vi "BMP180 Read.vi"(8 "error in (no error)":errorcluster, 9 "BMP180 Config":T1={"I2C"={"Slave Address"=64, "Channel"=0}, "Mode"=enum."Ultra Low Power", "Cal Coefs"={"AC1"={"Addr:"=170, "Val:"=0}, "AC2"={"Addr:"=172, "Val:"=0}, "AC3"={"Addr:"=174, "Val:"=0}, "AC4"={"Addr:"=176, "Val:"=0}, "AC5"={"Addr:"=178, "Val:"=0}, "AC6"={"Addr:"=180, "Val:"=0}, "B1"={"Addr:"=182, "Val:"=0}, "B2"={"Addr:"=184, "Val:"=0}, "MB"={"Addr:"=186, "Val:"=0}, "MC"={"Addr:"=188, "Val:"=0}, "MD"={"Addr:"=190, "Val:"=0}}, "Online"=FALSE} {"I2C"."Slave Address" format="%.0x"; "Cal Coefs"."MD"."Val:" format="%04x"; "Cal Coefs"."MD"."Addr:" format="%02x"; "Cal Coefs"."MC"."Val:" format="%04x"; "Cal Coefs"."MC"."Addr:" format="%02x"; "Cal Coefs"."MB"."Val:" format="%04x"; "Cal Coefs"."MB"."Addr:" format="%02x"; "Cal Coefs"."B2"."Val:" format="%04x"; "Cal Coefs"."B2"."Addr:" format="%02x"; "Cal Coefs"."B1"."Val:" format="%04x"; "Cal Coefs"."B1"."Addr:" format="%02x"; "Cal Coefs"."AC6"."Val:" format="%04x"; "Cal Coefs"."AC6"."Addr:" format="%02x"; "Cal Coefs"."AC5"."Val:" format="%04x"; "Cal Coefs"."AC5"."Addr:" format="%02x"; "Cal Coefs"."AC4"."Val:" format="%04x"; "Cal Coefs"."AC4"."Addr:" format="%02x"; "Cal Coefs"."AC3"."Val:" format="%04x"; "Cal Coefs"."AC3"."Addr:" format="%02x"; "Cal Coefs"."AC2"."Val:" format="%04x"; "Cal Coefs"."AC2"."Addr:" format="%02x"; "Cal Coefs"."AC1"."Val:" format="%04x"; "Cal Coefs"."AC1"."Addr:" format="%02x"}, 11 "LINX Resource in":T3) -> (0 "error out":errorcluster, 1 "BMP180 Config":T1={"I2C"={"Slave Address"=64, "Channel"=0}, "Mode"=enum."Ultra Low Power", "Cal Coefs"={"AC1"={"Addr:"=170, "Val:"=0}, "AC2"={"Addr:"=172, "Val:"=0}, "AC3"={"Addr:"=174, "Val:"=0}, "AC4"={"Addr:"=176, "Val:"=0}, "AC5"={"Addr:"=178, "Val:"=0}, "AC6"={"Addr:"=180, "Val:"=0}, "B1"={"Addr:"=182, "Val:"=0}, "B2"={"Addr:"=184, "Val:"=0}, "MB"={"Addr:"=186, "Val:"=0}, "MC"={"Addr:"=188, "Val:"=0}, "MD"={"Addr:"=190, "Val:"=0}}, "Online"=FALSE} {"I2C"."Slave Address" format="%.0x"; "Cal Coefs"."MD"."Val:" format="%04x"; "Cal Coefs"."MD"."Addr:" format="%02x"; "Cal Coefs"."MC"."Val:" format="%04x"; "Cal Coefs"."MC"."Addr:" format="%02x"; "Cal Coefs"."MB"."Val:" format="%04x"; "Cal Coefs"."MB"."Addr:" format="%02x"; "Cal Coefs"."B2"."Val:" format="%04x"; "Cal Coefs"."B2"."Addr:" format="%02x"; "Cal Coefs"."B1"."Val:" format="%04x"; "Cal Coefs"."B1"."Addr:" format="%02x"; "Cal Coefs"."AC6"."Val:" format="%04x"; "Cal Coefs"."AC6"."Addr:" format="%02x"; "Cal Coefs"."AC5"."Val:" format="%04x"; "Cal Coefs"."AC5"."Addr:" format="%02x"; "Cal Coefs"."AC4"."Val:" format="%04x"; "Cal Coefs"."AC4"."Addr:" format="%02x"; "Cal Coefs"."AC3"."Val:" format="%04x"; "Cal Coefs"."AC3"."Addr:" format="%02x"; "Cal Coefs"."AC2"."Val:" format="%04x"; "Cal Coefs"."AC2"."Addr:" format="%02x"; "Cal Coefs"."AC1"."Val:" format="%04x"; "Cal Coefs"."AC1"."Addr:" format="%02x"}, 2 "Pressure Reading":T2, 3 "LINX Resource":T3)   [LabVIEW 2018]
uses:
  Type Defs/pressureReading.ctl
  <vilib>/MakerHub/LINX/Private/Type Defs/Platform.ctl
  <vilib>/MakerHub/LINX/Private/Type Defs/Interface.ctl
  <vilib>/MakerHub/LINX/Private/Device/Type Defs/TCP Config.ctl
  <vilib>/MakerHub/LINX/Private/Device/Type Defs/Channels.ctl
  <vilib>/MakerHub/LINX/Private/Device/Type Defs/LINX Device Config.ctl
  <vilib>/MakerHub/LINX/Private/Type Defs/LINX Ref.ctl
  BMP180 Config Options.ctl
panel:
  out "Raw Pres":i32
  out "Raw Temp":i32
  out "B6":i32
  out "B7":u32
  out "B4":u32
  out "B3":i32
  out "B5":i32
  out "X3":i32
  out "X2":i32
  out "X1":i32
  # "These values are solely for checking work"
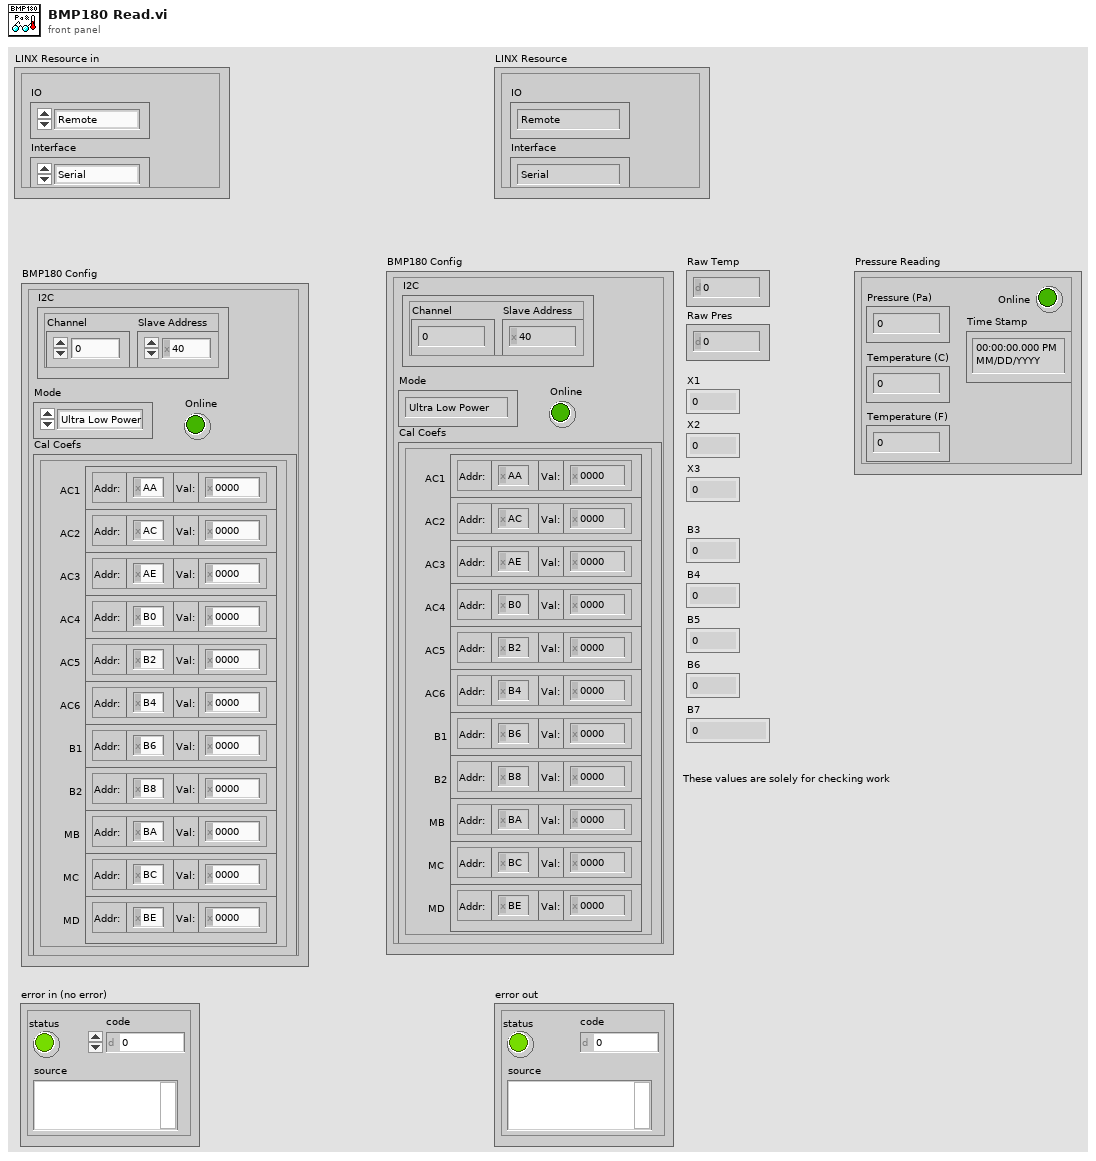
[diagram p1: front panel]
types:
  T1 = typedef "BMP180 Config Options.ctl" = cluster{"I2C":cluster{"Slave Address":u8, "Channel":u8}, "Mode":enum8{"Ultra Low Power", "Standard", "High Resolution", "Ultra High Resolution"}, "Cal Coefs":cluster{"AC1":cluster{"Addr:":u8, "Val:":u16}, "AC2":cluster{"Addr:":u8, "Val:":u16}, "AC3":cluster{"Addr:":u8, "Val:":u16}, "AC4":cluster{"Addr:":u8, "Val:":u16}, "AC5":cluster{"Addr:":u8, "Val:":u16}, "AC6":cluster{"Addr:":u8, "Val:":u16}, "B1":cluster{"Addr:":u8, "Val:":u16}, "B2":cluster{"Addr:":u8, "Val:":u16}, "MB":cluster{"Addr:":u8, "Val:":u16}, "MC":cluster{"Addr:":u8, "Val:":u16}, "MD":cluster{"Addr:":u8, "Val:":u16}}, "Online":bool}
  T2 = typedef "pressureReading.ctl" = cluster{"Time Stamp":timestamp, "Online":bool, "Temperature (C)":dbl, "Pressure (Pa)":dbl, "Temperature (F)":dbl}
  T3 = typedef "LMH-LINX.lvlib/LINX Ref.ctl" = cluster{"IO":T4, "Interface":T5, "LINX Device Config":T6}
  T4 = typedef "LMH-LINX.lvlib/Platform.ctl" = enum16{"Remote", "Local"}
  T5 = typedef "LMH-LINX.lvlib/Interface.ctl" = enum16{"Serial", "TCP"}
  T6 = typedef "LMH-LINX.lvlib/Device.lvlib/LINX Device Config.ctl" = cluster{"Interface":T5, "COM Port":refnum<visa-resource-name>, "TCP Configuration":T7, "Device Family":u8, "Device ID":u8, "Device Name":string, "TCP Ref":refnum<k5>, "Channels":T8}
  T7 = typedef "LMH-LINX.lvlib/Device.lvlib/TCP Config.ctl" = cluster{"IP Address":string, "Port":u16}
  T8 = typedef "LMH-LINX.lvlib/Channels.ctl" = cluster{"DI":u8[], "DO":u8[], "AI":u8[], "AO":u8[], "PWM":u8[], "QE":u8[], "UART":u8[], "I2C 2":u8[], "SPI":u8[], "CAN":u8[], "Servo":u8[], "AI Ref (V)":dbl, "AI Resolution (Bits)":u8, "AO Ref (V)":dbl, "AO Resolution (Bits)":u8}
  T9 = enum8{"Ultra Low Power", "Standard", "High Resolution", "Ultra High Resolution"}
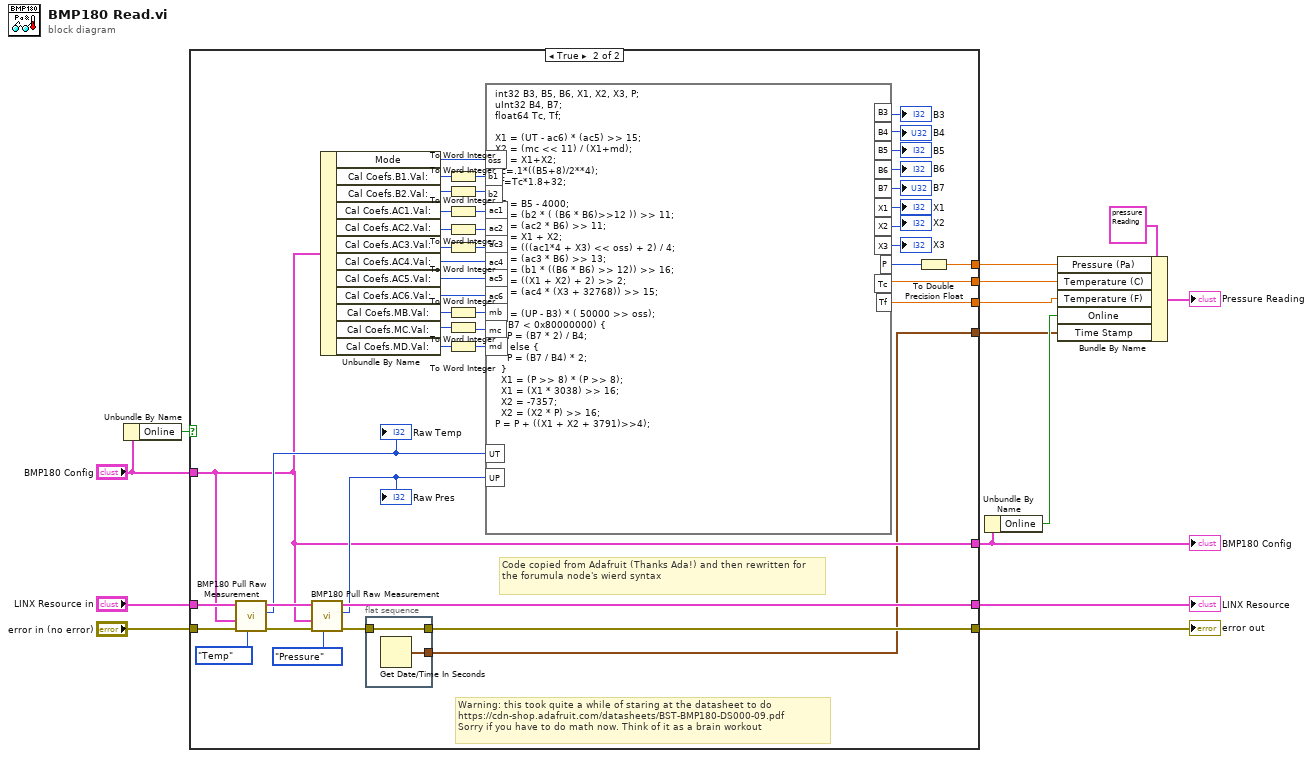
[diagram p0: block diagram]
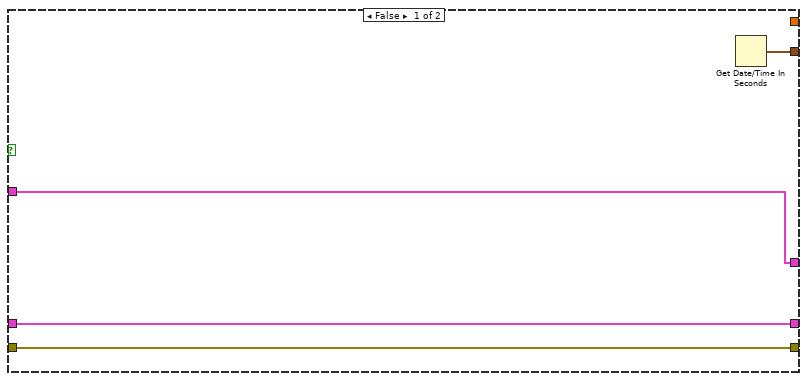
[diagram p2: hidden frame]
diagram:
  n1 = Unbundle By Name("BMP180 Config") -> ("Online"=w9:bool)
  n2 = case shown="True" w9 {
    tunnel: "error in (no error)" -> [w17 w63]
    tunnel: "LINX Resource in" -> [w18 w62]
    tunnel: [w18 w58] -> w12
    tunnel: [w17 w25] -> w11
    tunnel: "BMP180 Config" -> [w15 w24]
    tunnel: [w15 w24] -> w6
    tunnel: [_ w22] -> w7
    tunnel: [_ w21] -> w4
    tunnel: [_ w20] -> w3
    tunnel: [w16 w19] -> w2
    frame False {
      n3 = Get Date/Time In Seconds() -> (seconds since 1Jan1904=w16:timestamp)
    }
    frame True {
      # "Code copied from Adafruit (Thanks Ada!) and then rewritten for the forumula node's wierd syntax"
      # "Warning: this took quite a while of staring at the datasheet to do\nhttps://cdn-shop.adafruit.com/datasheets/BST-BMP180-DS000-09.pdf\nSorry if you have to do math now. Think of it as a brain workout"
      n4 = call "BMP180 Pull Raw Measurement.vi"("Sensor Type"=enum16{"Temp", "Pressure"}."Temp", "error in (no error)"=w63, "BMP180 Config"=w24, "LINX Resource in"=w62) -> ("error out"=w59:errorcluster, "Raw Reading"=w28:i32, "LINX Resource"=w60:T3)  [unwired: 5 in]
      "Raw Temp" <- w28
      n5 = call "BMP180 Pull Raw Measurement.vi"("Sensor Type"=enum16{"Temp", "Pressure"}."Pressure", "error in (no error)"=w59, "BMP180 Config"=w24, "LINX Resource in"=w60) -> ("error out"=w26:errorcluster, "Raw Reading"=w27:i32, "LINX Resource"=w58:T3)  [unwired: 5 in]
      "Raw Pres" <- w27
      n6 = Unbundle By Name(w24) -> ("Mode"=w45:T9, "Cal Coefs.B1.Val:"=w46:u16, "Cal Coefs.B2.Val:"=w43:u16, "Cal Coefs.AC1.Val:"=w42:u16, "Cal Coefs.AC2.Val:"=w41:u16, "Cal Coefs.AC3.Val:"=w40:u16, "Cal Coefs.AC4.Val:"=w39:u16, "Cal Coefs.AC5.Val:"=w38:u16, "Cal Coefs.AC6.Val:"=w37:u16, "Cal Coefs.MB.Val:"=w48:u16, "Cal Coefs.MC.Val:"=w34:u16, "Cal Coefs.MD.Val:"=w47:u16)
      n7 = flat-sequence {
        tunnel: w26 -> [w65]
        tunnel: [w65] -> w25
        tunnel: [w64] -> w19
        frame #0 {
          n8 = Get Date/Time In Seconds() -> (seconds since 1Jan1904=w64:timestamp)
        }
      }
      n9 = To Word Integer(number=w46) -> (16bit integer=w44:i16)
      n10 = To Word Integer(number=w43) -> (16bit integer=w52:i16)
      n11 = To Word Integer(number=w42) -> (16bit integer=w51:i16)
      n12 = To Word Integer(number=w41) -> (16bit integer=w50:i16)
      n13 = To Word Integer(number=w40) -> (16bit integer=w49:i16)
      n14 = To Word Integer(number=w48) -> (16bit integer=w36:i16)
      n15 = To Word Integer(number=w34) -> (16bit integer=w35:i16)
      n16 = To Word Integer(number=w47) -> (16bit integer=w33:i16)
      n17 = formula code="int32 B3, B5, B6, X1, X2, X3, P;\nuInt32 B4, B7;\nfloat64 Tc, Tf;\n\nX1 = (UT - ac6) * (ac5) >> 15;\nX2 = (mc << 11) / (X1+md);\nB5 = X1+X2;\nTc=.1*((B5+8)/2**4);\nTf=Tc*1.8+32;\n\nB6 = B5 - 4000;\nX1 = (b2 * ( (B6 * B6)>>12 )) >> 11;\nX2 = (ac2 * B6) >> 11;\nX3 = X1 + X2;\nB3 = (((ac1*4 + X3) << oss) + 2) / 4;\nX1 = (ac3 * B6) >> 13;\nX2 = (b1 * ((B6 * B6) >> 12)) >> 16;\nX3 = ((X1 + X2) + 2) >> 2;\nB4 = (ac4 * (X3 + 32768)) >> 15;\n  \nB7 = (UP - B3) * ( 50000 >> oss);\nif (B7 < 0x80000000) {\n    P = (B7 * 2) / B4;\n  } else {\n    P = (B7 / B4) * 2;\n  }\n  X1 = (P >> 8) * (P >> 8);\n  X1 = (X1 * 3038) >> 16;\n  X2 = -7357; \n  X2 = (X2 * P) >> 16;\nP = P + ((X1 + X2 + 3791)>>4);"("UT"=w28, "ac1"=w51, "ac2"=w50, "ac3"=w49, "ac4"=w39, "b2"=w52, "b1"=w44, "oss"=w45, "UP"=w27, "ac5"=w38, "ac6"=w37, "mb"=w36, "mc"=w35, "md"=w33) -> ("P"=w23:i32, "X1"=→"X1":i32, "X2"=→"X2":i32, "B5"=→"B5":i32, "B3"=→"B3":i32, "B4"=→"B4":u32, "B6"=→"B6":i32, "X3"=→"X3":i32, "Tc"=w21:dbl, "B7"=→"B7":u32, "Tf"=w20:dbl)
      n18 = To Double Precision Float(number=w23) -> (double precision float=w22:dbl)
    }
  }
  "error out" <- w11
  "LINX Resource" <- w12
  "BMP180 Config" <- w6
  n19 = Unbundle By Name(w6) -> ("Online"=w5:bool)
  n20 = Bundle By Name(cluster=T2 {"Time Stamp"=timestamp(0 s since 1904-01-01), "Online"=FALSE, "Temperature (C)"=0.0, "Pressure (Pa)"=0.0, "Temperature (F)"=0.0} ("Pressure Reading"), "Pressure (Pa)"=w7, "Temperature (C)"=w4, "Temperature (F)"=w3, "Online"=w5, "Time Stamp"=w2) -> (→"Pressure Reading":T2)
